vi "TEST - LVOOP Get Default Object.vi"(8 "error in (no error)":errorcluster) -> (0 "error out":errorcluster, 2 "Pass":bool)   [LabVIEW 2013]
uses:
  LVOOP Data/Class 1/Class 1.lvclass
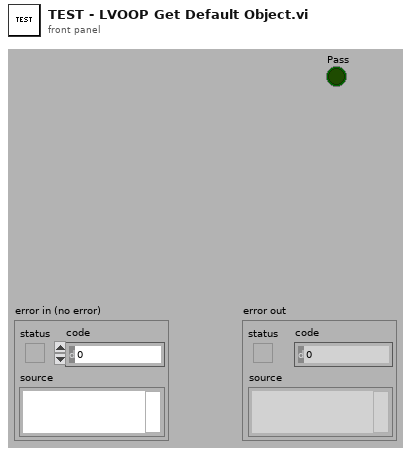
[diagram p1: front panel]
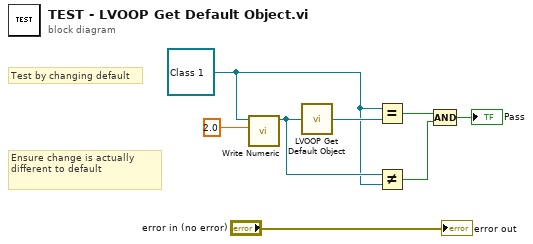
[diagram p0: block diagram]
diagram:
  w1 = refnum<class "Class 1.lvclass"> refnum ("Class 1.lvclass")
  # "Ensure change is actually different to default"
  # "Test by changing default"
  n1 = call "Write Numeric.vi"("Numeric"=2.0, "Class 1 in"=w1) -> ("Class 1 out"=w2:refnum<class "Class 1.lvclass">)  [unwired: 9 in]
  n2 = call "LVOOP Get Default Object.vi"("Object"=w2) -> ("Object Default Instance"=w5:refnum<class "Class 1.lvclass">)
  n3 = Equal?(x=w1, y=w5) -> (x = y?=w4:bool)
  n4 = Not Equal?(x=w2, y=w1) -> (x != y?=w3:bool)
  n5 = Compound Arithmetic op=AND(w4, w3) -> (→"Pass":bool)
  "error out" <- "error in (no error)"
